vi "4bar encoder to angle.vi"(1 "Encoder Position":dbl) -> (0 "4bar Angle Radians":dbl)   [LabVIEW 2018]
panel:
  # "make 0 be horizantal"
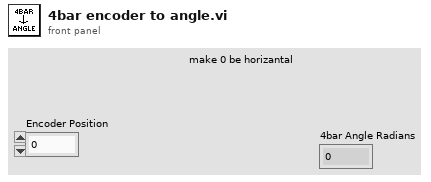
[diagram p1: front panel]
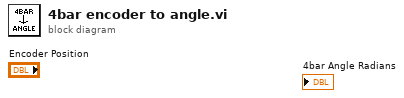
[diagram p0: block diagram]
diagram:
